vi "Servo Acceleration.vi"(4 "Angle get":u16) -> (1 "Angle Set":i32)   [LabVIEW 2012]
uses:
  <vilib>/addons/control/pid/NI_PID_pid.lvlib
  <vilib>/addons/control/pid/pid.llb/PID Control Input Filter (DBL).vi
panel:
  in  "reinitialize? (F)":bool
  out "Array":u16[](array[numeric])
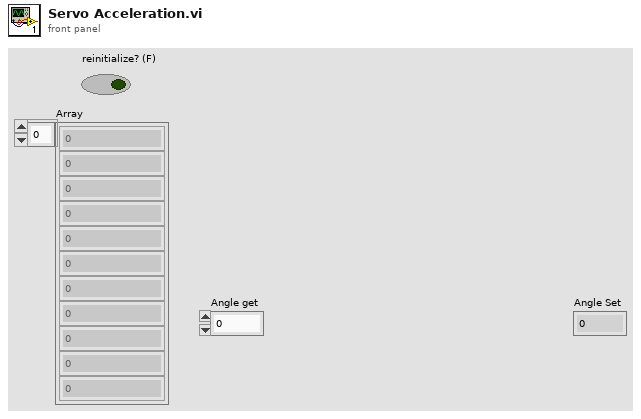
[diagram p1: front panel]
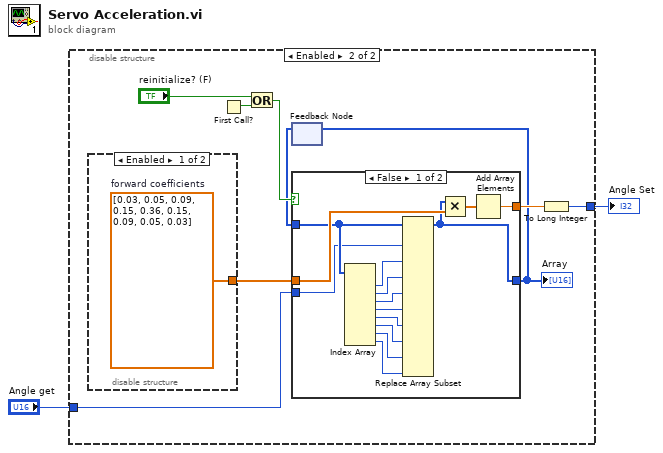
[diagram p0: block diagram]
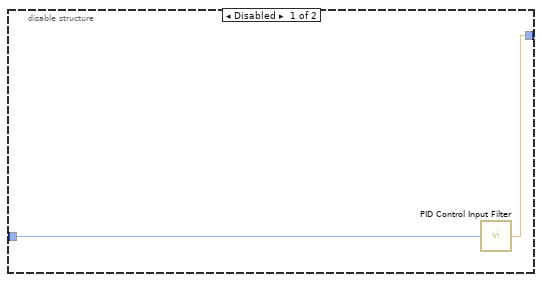
[diagram p2: hidden frame]
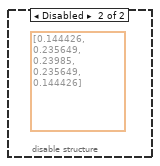
[diagram p3: hidden frame]
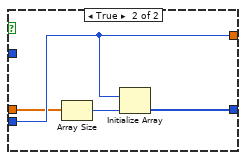
[diagram p4: hidden frame]
diagram:
  n1 = disable-structure shown="Enabled" {
    disable-tunnel: "Angle get" -> [w4 w10]
    disable-tunnel: [w3 w5] -> w1
    frame Disabled {
      n2 = call-poly <vilib>:"PID Control Input Filter.vi"("input"=w4) -> ("output"=w3:dbl)  [unwired: 1 in, 3 out]
    }
    frame Enabled {
      n3 = disable-structure shown="Enabled" {
        disable-tunnel: [w14 _] -> w6
        frame Enabled {
          w14 = dbl[] [0.03, 0.05, 0.09, 0.15, 0.36, 0.15, 0.09, 0.05, 0.03]  # forward coefficients
        }
        frame Disabled {
          (unwired) dbl[] [0.144426, 0.235649, 0.23985, 0.235649, 0.144426] ("forward coefficients 2")
        }
      }
      n4 = First Call?() -> (First Call?: T/F=w11:bool)
      n5 = Or(x="reinitialize? (F)", y=w11) -> (x .or. y?=w13:bool)
      n6 = feedback #1() -> (w7:u16[])  [unwired: 1 in]
      n7 = case shown="False" w13 {
        tunnel: w6 -> [w28 w29]
        tunnel: w7 -> [w25 _]
        tunnel: [w27 w30] -> w9
        tunnel: [w19 w31] -> w8
        tunnel: w10 -> [w24 w30]
        frame False {
          n8 = Index Array(array=w25) -> (element #1=w23:u16, element #2=w22:u16, element #3=w21:u16, element #4=w20:u16, element #5=w18:u16, element #6=w17:u16, element #7=w16:u16, element #8=w15:u16)  [unwired: 8 in]
          n9 = Replace Array Subset(array=w25, new element #1=w24, new element #2=w23, new element #3=w22, new element #4=w21, new element #5=w20, new element #6=w18, new element #7=w17, new element #8=w16, new element #9=w15) -> (w19:u16[])  [unwired: 9 in]
          n10 = Multiply(x=w19, y=w28) -> (x*y=w26:dbl[])
          n11 = Add Array Elements(numeric array=w26) -> (sum=w27:dbl)
        }
        frame True {
          n12 = Array Size(array=w29) -> (size(s)=w32:i32)
          n13 = Initialize Array(w30, w32) -> (w31:u16[])
        }
      }
      "Array" <- w8
      n14 = feedback-in #1(w8) -> ()
      n15 = To Long Integer(number=w9) -> (32bit integer=w5:i32)
    }
  }
  "Angle Set" <- w1
